vi "unpack Galvo data-test.vi"() -> ()   [LabVIEW 2015]
panel:
  in  "stop":bool
  out "Galvo signal out":u32
  out "output valid?":bool
  out "packer out":T1
  in  "packer in":T1
  out "Galvo index out":T2(ring)
  in  "input valid?":bool
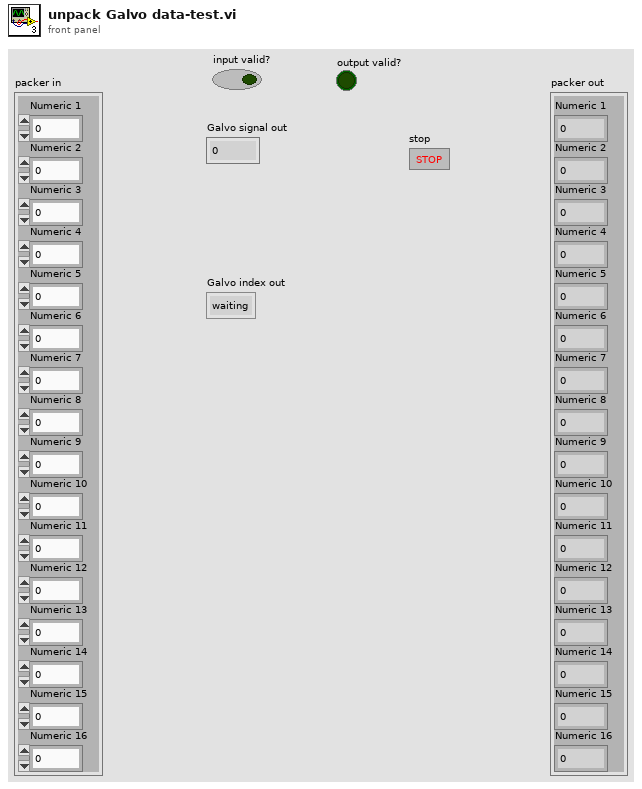
[diagram p1: front panel]
types:
  T1 = cluster{"Numeric 1":u32, "Numeric 2":u32, "Numeric 3":u32, "Numeric 4":u32, "Numeric 5":u32, "Numeric 6":u32, "Numeric 7":u32, "Numeric 8":u32, "Numeric 9":u32, "Numeric 10":u32, "Numeric 11":u32, "Numeric 12":u32, "Numeric 13":u32, "Numeric 14":u32, "Numeric 15":u32, "Numeric 16":u32}
  T2 = enum16{"waiting", "Numeric 1", "Numeric 2", "Numeric 3", "Numeric 4", "Numeric 5", "Numeric 6", "Numeric 7", "Numeric 8", "Numeric 9", "Numeric 10", "Numeric 11", "Numeric 12", "Numeric 13", "Numeric 14", "Numeric 15", "Numeric 16"}
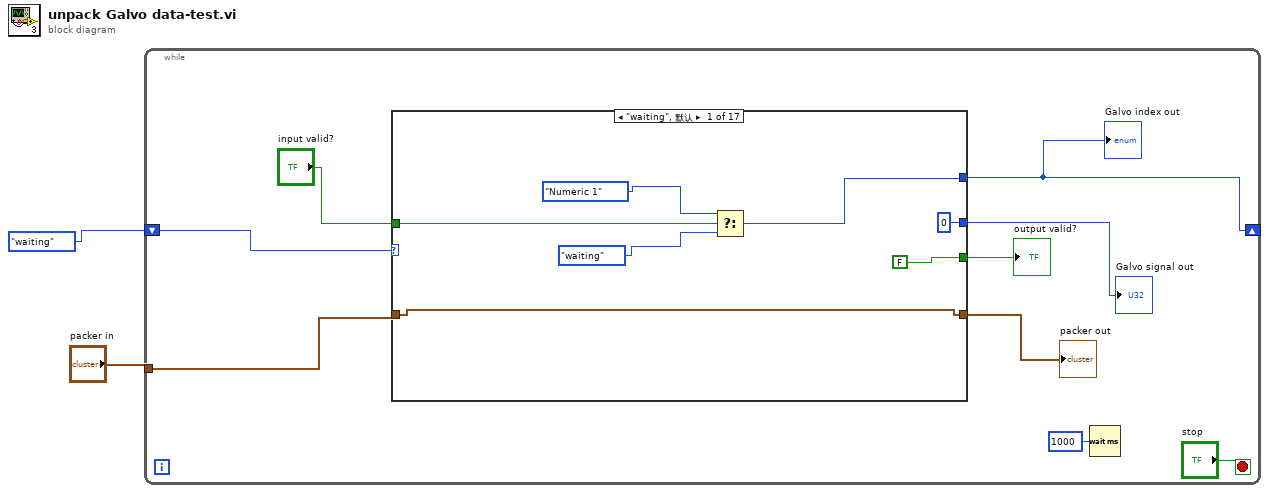
[diagram p0: block diagram]
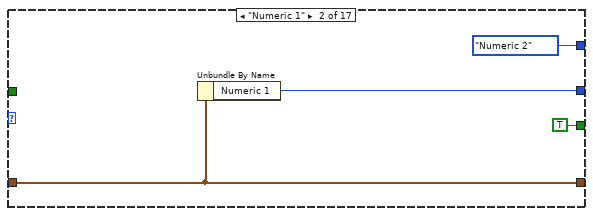
[diagram p2: hidden frame]
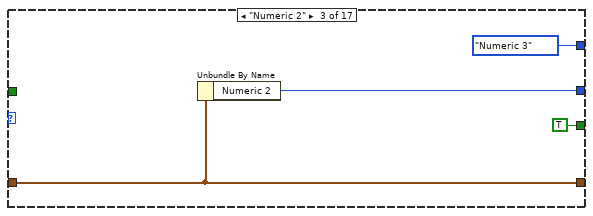
[diagram p3: hidden frame]
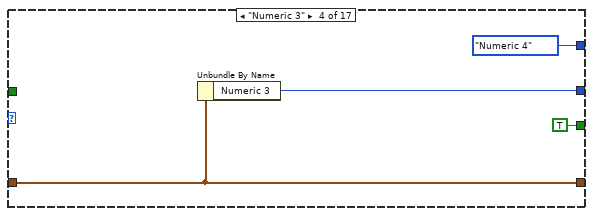
[diagram p4: hidden frame]
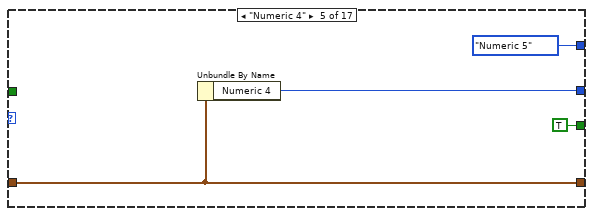
[diagram p5: hidden frame]
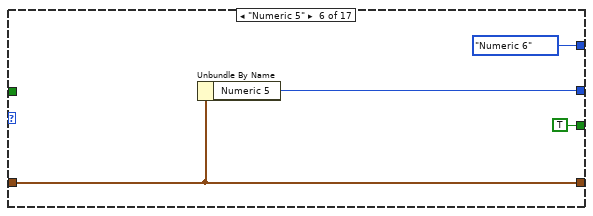
[diagram p6: hidden frame]
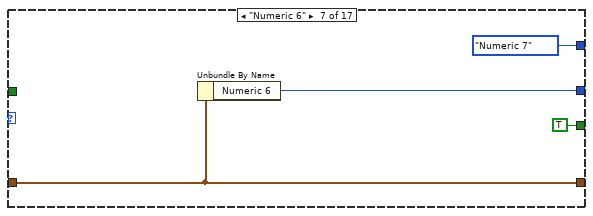
[diagram p7: hidden frame]
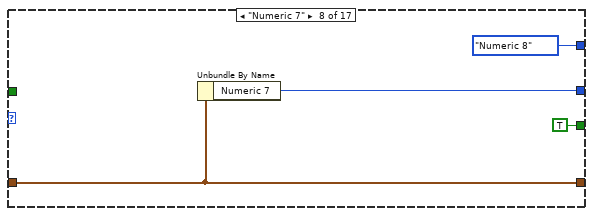
[diagram p8: hidden frame]
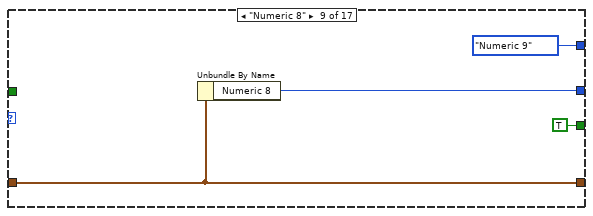
[diagram p9: hidden frame]
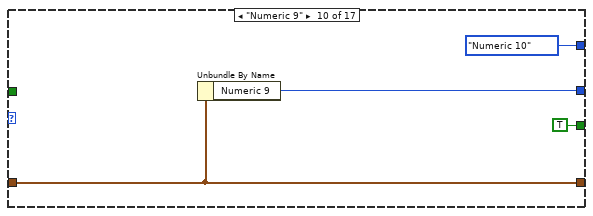
[diagram p10: hidden frame]
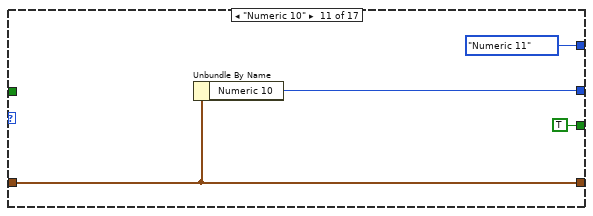
[diagram p11: hidden frame]
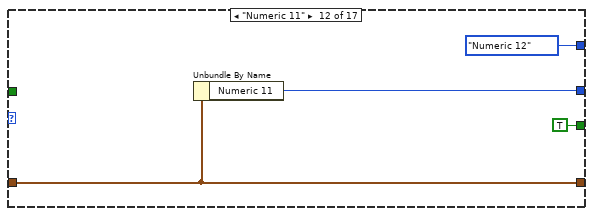
[diagram p12: hidden frame]
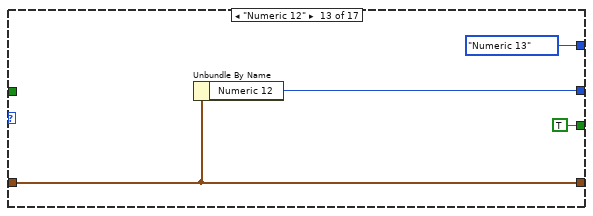
[diagram p13: hidden frame]
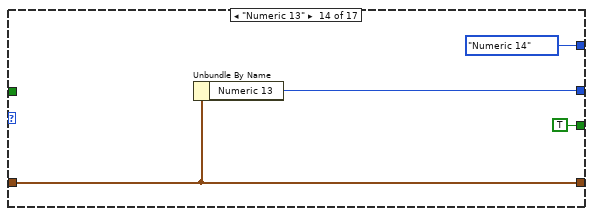
[diagram p14: hidden frame]
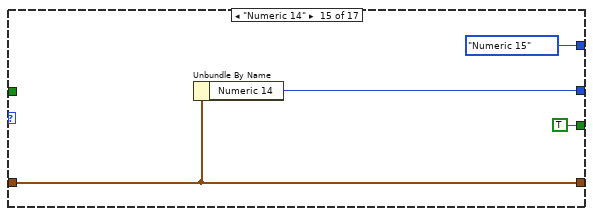
[diagram p15: hidden frame]
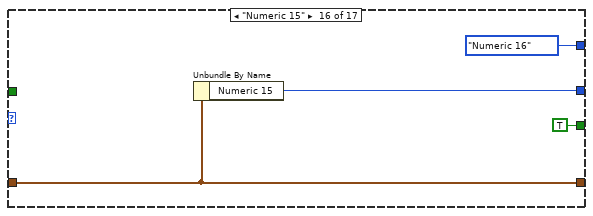
[diagram p16: hidden frame]
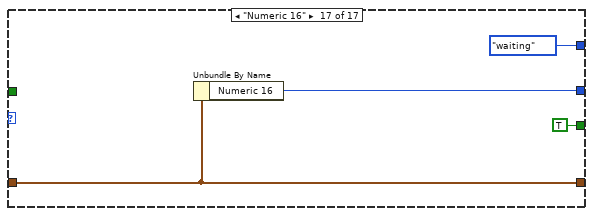
[diagram p17: hidden frame]
diagram:
  n1 = while {
    tunnel: "packer in" -> [w10]
    shift-right: [w5] -> _
    shift-left: T2."waiting" ("Galvo index in") -> [w6]
    stop <- "stop" stop-if-true
    n2 = case shown="\"waiting\", 默认" w6 {
      tunnel: "input valid?" -> [w18 _ _ _ _ _ _ _ _ _ _ _ _ _ _ _ _]
      tunnel: w10 -> [w13 w19 w23 w27 w31 w35 w39 w43 w47 w51 w55 w59 w63 w67 w71 w75 w79]
      tunnel: [w17 T2."Numeric 2" ("Galvo index in") T2."Numeric 3" ("Galvo index in") T2."Numeric 4" ("Galvo index in") T2."Numeric 5" ("Galvo index in") T2."Numeric 6" ("Galvo index in") T2."Numeric 7" ("Galvo index in") T2."Numeric 8" ("Galvo index in") T2."Numeric 9" ("Galvo index in") T2."Numeric 10" ("Galvo index in") T2."Numeric 11" ("Galvo index in") T2."Numeric 12" ("Galvo index in") T2."Numeric 13" ("Galvo index in") T2."Numeric 14" ("Galvo index in") T2."Numeric 15" ("Galvo index in") T2."Numeric 16" ("Galvo index in") T2."waiting" ("Galvo index in")] -> w5
      tunnel: [FALSE TRUE TRUE TRUE TRUE TRUE TRUE TRUE TRUE TRUE TRUE TRUE TRUE TRUE TRUE TRUE TRUE] -> w9
      tunnel: [u32 0 ("Numeric 3") w20 w24 w28 w32 w36 w40 w44 w48 w52 w56 w60 w64 w68 w72 w76 w80] -> w8
      tunnel: [w13 w19 w23 w27 w31 w35 w39 w43 w47 w51 w55 w59 w63 w67 w71 w75 w79] -> w7
      frame "waiting", Default {
        n3 = Select(t=T2."Numeric 1" ("Galvo index in"), s=w18, f=T2."waiting" ("Galvo index in")) -> (s? t:f=w17:T2)
      }
      frame "Numeric 1" {
        n4 = Unbundle By Name(w19) -> ("Numeric 1"=w20:u32)
      }
      frame "Numeric 2" {
        n5 = Unbundle By Name(w23) -> ("Numeric 2"=w24:u32)
      }
      frame "Numeric 3" {
        n6 = Unbundle By Name(w27) -> ("Numeric 3"=w28:u32)
      }
      frame "Numeric 4" {
        n7 = Unbundle By Name(w31) -> ("Numeric 4"=w32:u32)
      }
      frame "Numeric 5" {
        n8 = Unbundle By Name(w35) -> ("Numeric 5"=w36:u32)
      }
      frame "Numeric 6" {
        n9 = Unbundle By Name(w39) -> ("Numeric 6"=w40:u32)
      }
      frame "Numeric 7" {
        n10 = Unbundle By Name(w43) -> ("Numeric 7"=w44:u32)
      }
      frame "Numeric 8" {
        n11 = Unbundle By Name(w47) -> ("Numeric 8"=w48:u32)
      }
      frame "Numeric 9" {
        n12 = Unbundle By Name(w51) -> ("Numeric 9"=w52:u32)
      }
      frame "Numeric 10" {
        n13 = Unbundle By Name(w55) -> ("Numeric 10"=w56:u32)
      }
      frame "Numeric 11" {
        n14 = Unbundle By Name(w59) -> ("Numeric 11"=w60:u32)
      }
      frame "Numeric 12" {
        n15 = Unbundle By Name(w63) -> ("Numeric 12"=w64:u32)
      }
      frame "Numeric 13" {
        n16 = Unbundle By Name(w67) -> ("Numeric 13"=w68:u32)
      }
      frame "Numeric 14" {
        n17 = Unbundle By Name(w71) -> ("Numeric 14"=w72:u32)
      }
      frame "Numeric 15" {
        n18 = Unbundle By Name(w75) -> ("Numeric 15"=w76:u32)
      }
      frame "Numeric 16" {
        n19 = Unbundle By Name(w79) -> ("Numeric 16"=w80:u32)
      }
    }
    "Galvo index out" <- w5
    "packer out" <- w7
    "output valid?" <- w9
    "Galvo signal out" <- w8
    n20 = Wait (ms)(milliseconds to wait=u32 1000) -> ()  [unwired: 1 out]
  }
